vi "Add Callback.vi"(7 "Owner":refnum<class>, 8 "error in (no error)":errorcluster, 10 "Callback":refnum<vi>, 11 "Callback Producer in":refnum<class "Callback Producer.lvclass">) -> (0 "error out":errorcluster, 3 "Callback Producer out":refnum<class "Callback Producer.lvclass">)   [LabVIEW 2020, in "Callback Producer.lvclass"]
uses:
  Callback Producer.lvclass
  Callback.ctl
  Callback Producer.lvclass/Callback Producer.ctl
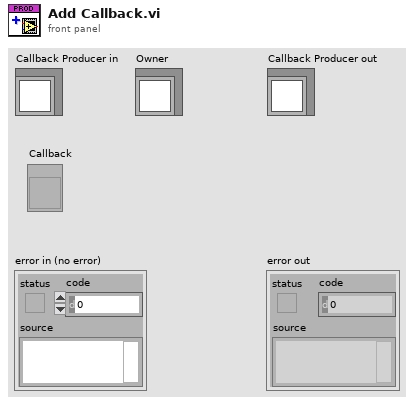
[diagram p1: front panel]
types:
  T1 = typedef "Callback Producer.lvclass/Callback.ctl" = cluster{"Owner":refnum<class>, "VI":refnum<vi>}
  T2 = typedef "Callback Producer.lvclass/Ref Data.ctl" = cluster{"Callbacks":T1[]}
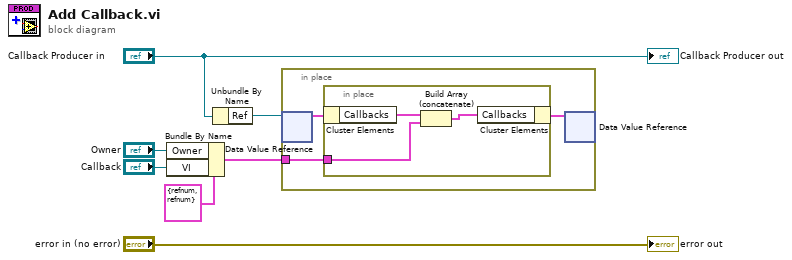
[diagram p0: block diagram]
diagram:
  n1 = Bundle By Name(cluster=T1 {"Owner"=refnum, "VI"=refnum} ("Callback"), "Owner"="Owner", "VI"="Callback") -> (w1:T1)
  n2 = Unbundle By Name("Callback Producer in") -> ("Ref"=w3:refnum<data-value>)
  n3 = in-place {
    in-place-border: w1 -> [w8]
    n4 = in-place-dvr #1(w3) -> (w10:T2)  [unwired: 1 out]
    n5 = in-place {
      in-place-border: w8 -> [w11]
      n6 = in-place-cluster #2(w10) -> ("Callbacks"=w13:T1[])
      n7 = Build Array (concatenate)(w13, w11) -> (w12:T1[])
      n8 = in-place-cluster #2("Callbacks"=w12) -> (w9:T2)
    }
    n9 = in-place-dvr #1(w9) -> ()  [unwired: 2 out]
  }
  "error out" <- "error in (no error)"
  "Callback Producer out" <- "Callback Producer in"
